vi "Test Serialize Arrays.vi"(8 "error in (no error)":errorcluster) -> (0 "error out":errorcluster)   [LabVIEW 2013]
uses:
  src/Serializer/JSON Serializer/JSON Serializer.lvclass
  <vilib>/addons/_JKI Toolkits/Caraya/classes/Test/Test.lvclass
  <vilib>/addons/_JKI Toolkits/Caraya/classes/Assert/Assert.lvclass
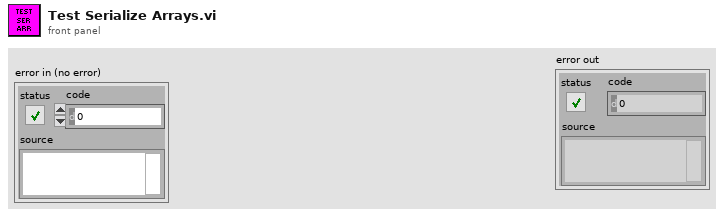
[diagram p1: front panel]
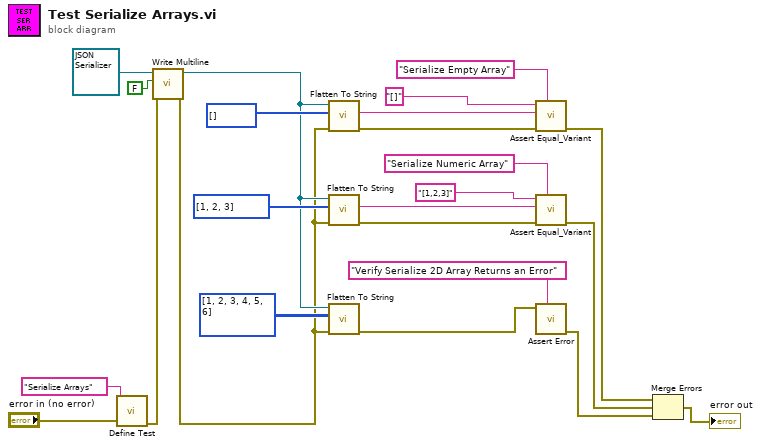
[diagram p0: block diagram]
diagram:
  n1 = call <vilib>:"Define Test.vi"("error in (no error)"="error in (no error)", "Label (VI Title)"="Serialize Arrays") -> ("error out"=w5:errorcluster)  [unwired: 9 in]
  n2 = call-dynamic "Write Multiline.vi"("error in (no error)"=w5, "Multiline"=FALSE, "JSON Serializer in"=refnum<class "JSON Serializer.lvclass"> refnum ("JKI JSON Serialization.lvlib:JSON Serializer.lvclass")) -> ("error out"=w1:errorcluster, "JSON Serializer out"=w6:refnum<class "JSON Serializer.lvclass">)  [unwired: 7 in]
  n3 = call-dynamic "Flatten To String.vi"("error in (no error)"=w1, "Variant"=i32[] [], "JSON Serializer in"=w6) -> ("error out"=w18:errorcluster, "String"=w17:string)  [unwired: 6 in, 1 out]
  n4 = call-dynamic "Flatten To String.vi"("error in (no error)"=w1, "Variant"=i32[] [1, 2, 3], "JSON Serializer in"=w6) -> ("error out"=w22:errorcluster, "String"=w21:string)  [unwired: 6 in, 1 out]
  n5 = call-dynamic "Flatten To String.vi"("error in (no error)"=w1, "Variant"=i32[][] [[1, 2, 3], [4, 5, 6]], "JSON Serializer in"=w6) -> ("error out"=w2:errorcluster)  [unwired: 6 in, 2 out]
  n6 = call <vilib>:"Assert Equal_Variant.vi"("Label"="Serialize Empty Array", "error in (no error)"=w18, "Y"=w17, "X"="[]") -> ("error out"=w11:errorcluster)  [unwired: 7 in]
  n7 = call <vilib>:"Assert Equal_Variant.vi"("Label"="Serialize Numeric Array", "error in (no error)"=w22, "Y"=w21, "X"="[1,2,3]") -> ("error out"=w12:errorcluster)  [unwired: 7 in]
  n8 = call <vilib>:"Assert Error.vi"("Label"="Verify Serialize 2D Array Returns an Error", "Error?"=w2) -> ("error out"=w13:errorcluster)  [unwired: 9 in]
  n9 = Merge Errors(w11, w12, w13) -> (→"error out":errorcluster)
